vi "Data - relative_file_path_handling.vi"(8 "error in":errorcluster, 11 "path in":path) -> (0 "error out":errorcluster, 3 "path out":path)   [LabVIEW 2019]
doc: "This is the general vi used to strip input file path to get the folder path that leads to that component based upon the type of enviroment the VI is running in\n1. LabVIEW development enviroment\n\n2. stand-alone application\n\nChenny Wang\n01/09/2007"
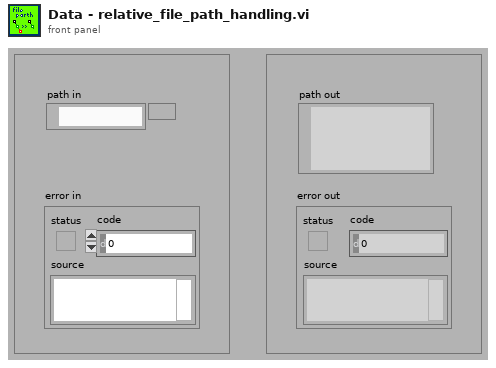
[diagram p1: front panel]
types:
  T1 = enum32{"invalid app kind", "Development System", "Run Time System", "Student Edition", "Embedded LabVIEW", "Evaluation", "Custom"}
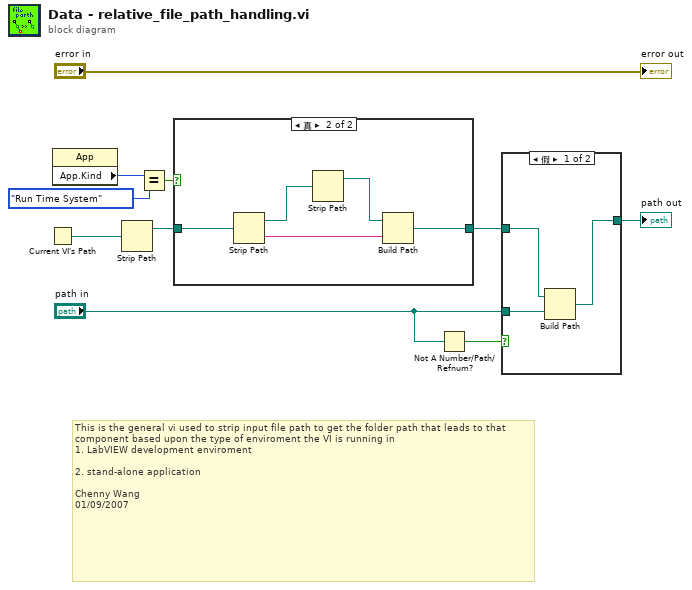
[diagram p0: block diagram]
diagram:
  # "This is the general vi used to strip input file path to get the folder path that leads to that component based upon the type of enviroment the VI is running in\n1. LabVIEW development enviroment\n\n2. stand-alone application\n\nChenny Wang\n01/09/2007"
  n1 = Current VI's Path() -> (path=w3:path)
  n2 = property class="App"() -> ("App.Kind"=w6:T1)  [unwired: 2 in, 2 out]
  n3 = Strip Path(path=w3) -> (stripped path=w2:path)  [unwired: 1 out]
  n4 = Equal?(x=w6, y=T1."Run Time System") -> (x = y?=w4:bool)
  n5 = case shown="真" w4 {
    tunnel: w2 -> [w11 w16]
    tunnel: [w11 w13] -> w1
    frame False {
    }
    frame True {
      n6 = Strip Path(path=w16) -> (stripped path=w12:path, name=w14:string)
      n7 = Strip Path(path=w12) -> (stripped path=w15:path)  [unwired: 1 out]
      n8 = Build Path(base path=w15, name or relative path=w14) -> (appended path=w13:path)
    }
  }
  n9 = Not A Number/Path/Refnum?(number/path/refnum="path in") -> (NaN/Path/Refnum?=w10:bool)
  n10 = case shown="假" w10 {
    tunnel: w1 -> [w19 w20]
    tunnel: "path in" -> [w18 _]
    tunnel: [w17 w20] -> w8
    frame False {
      n11 = Build Path(base path=w19, name or relative path=w18) -> (appended path=w17:path)
    }
    frame True {
    }
  }
  "path out" <- w8
  "error out" <- "error in"
